vi "RUSHHarvester.vi"(0 "Balls In Robot":i32, 1 "Speed of Harvester":dbl, 5 "Shoot":bool, 7 "Ball S12 Process":bool, 9 "Ball S3 Process":bool, 11 "Speed of Conveyor":dbl, 12 "SP 1 Triggered":bool, 13 "SP 2 Triggered":bool, 14 "SP 3 Triggered":bool) -> (2 "Conveyer Output":dbl, 3 "Harvester Output":dbl, 4 "Balls In Robot Output":i32, 6 "Shoot Output":bool, 8 "Ball S12 Process Output":bool, 10 "Ball S3 Process Output":bool)   [LabVIEW 2011]
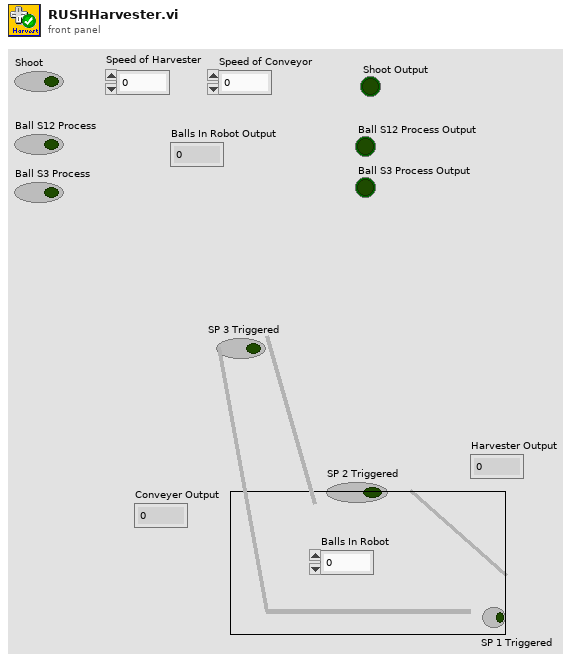
[diagram p1: front panel]
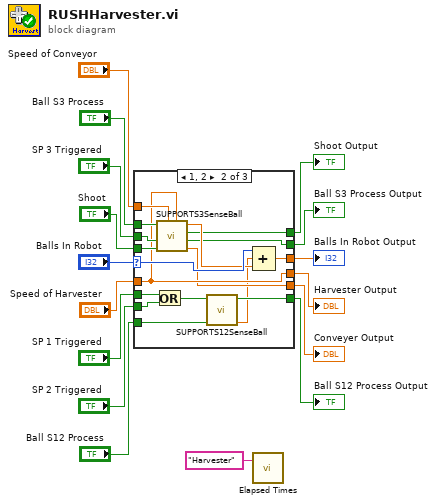
[diagram p0: block diagram]
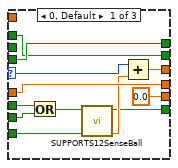
[diagram p2: hidden frame]
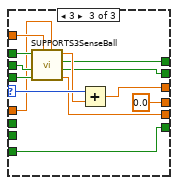
[diagram p3: hidden frame]
diagram:
  n1 = case shown="1, 2" "Balls In Robot" {
    selector: "Balls In Robot" -> [w27 w42 w57]
    tunnel: "SP 1 Triggered" -> [w25 w44 _]
    tunnel: "SP 2 Triggered" -> [w24 w45 _]
    tunnel: [w28 w37 0.0 ("Speed of Harvester")] -> w16
    tunnel: "Speed of Harvester" -> [w28 w37 w50]
    tunnel: "Speed of Conveyor" -> [_ w38 w51]
    tunnel: [0.0 ("Conveyer Output") w33 w46] -> w4
    tunnel: [w26 w43 w56] -> w3
    tunnel: "SP 3 Triggered" -> [_ w40 w53]
    tunnel: "Ball S3 Process" -> [w22 w39 w52]
    tunnel: "Ball S12 Process" -> [w20 w31 w55]
    tunnel: [w17 w30 w55] -> w5
    tunnel: "Shoot" -> [w23 w41 w54]
    tunnel: [w23 w35 w48] -> w6
    tunnel: [w22 w34 w47] -> w2
    frame 0, Default {
      n2 = Or(x=w25, y=w24) -> (x .or. y?=w19:bool)
      n3 = call "SUPPORTS12SenseBall.vi"("Ball in Process in"=w20, "Sense Ball"=w19) -> ("Ball Counter"=w18:dbl, "Ball in Process out"=w17:bool)  [unwired: 8 in]
      n4 = Add(x=w27, y=w18) -> (x+y=w26:dbl)
    }
    frame 1, 2 {
      n5 = Or(x=w44, y=w45) -> (x .or. y?=w32:bool)
      n6 = call "SUPPORTS3SenseBall.vi"("Harvester Speed"=w37, "Conveyor Speed"=w38, "Shoot"=w41, "Sense Ball"=w40, "Ball S3 Process"=w39) -> ("Conveyer Output"=w33:dbl, "Ball S3 Process Output"=w34:bool, "Shoot Output"=w35:bool, "Ball Counter"=w36:dbl)  [unwired: 3 in]
      n7 = call "SUPPORTS12SenseBall.vi"("Ball in Process in"=w31, "Sense Ball"=w32) -> ("Ball Counter"=w29:dbl, "Ball in Process out"=w30:bool)  [unwired: 8 in]
      n8 = Compound Arithmetic op=ADD(w42, w29, w36) -> (w43:dbl)
    }
    frame 3 {
      n9 = call "SUPPORTS3SenseBall.vi"("Harvester Speed"=w50, "Conveyor Speed"=w51, "Shoot"=w54, "Sense Ball"=w53, "Ball S3 Process"=w52) -> ("Conveyer Output"=w46:dbl, "Ball S3 Process Output"=w47:bool, "Shoot Output"=w48:bool, "Ball Counter"=w49:dbl)  [unwired: 3 in]
      n10 = Add(x=w57, y=w49) -> (x+y=w56:dbl)
    }
  }
  "Shoot Output" <- w6
  "Ball S12 Process Output" <- w5
  "Harvester Output" <- w16
  "Conveyer Output" <- w4
  "Balls In Robot Output" <- w3
  "Ball S3 Process Output" <- w2
  n11 = call "Elapsed Times.vi"("Call Name"="Harvester") -> ()  [unwired: 2 in, 1 out]
